vi "DG Measure.vi"(5 "PJVS setup":T2={"PJVS type"=enum."AC-supraVOLTcontrol", "Status Refnum"=refnum, "AC-supraVOLTcontrol"={"IP address:port (0.0.0.0:0000)"="0.0.0.0:0000", "Timeouts"={"TCP Read & Write (ms)"=7000, "Sensors readout"=5000, "PJVS setup"=10000, "Nullmeter readout"=5000, "Multiplexer setup"=3000, "57XX setup"=15000, "Generator setup"=5000, "Synthesizer setup"=3000, "Sampler readout"=10000}, "Simulation mode"=FALSE, "Debug mode"=FALSE}, "NPL bias source"={"DataSocketCluster"={"Server Machine"="CZC", "Client Machine"="localhost", "Data"="P2", "TimeStamp"=0.0, "Count"=1, "Target Process"="General Server"}}, "Manual PJVS"={"PJVS frequency (Hz)"=0.0, "Reference voltages (V)"=[], "File with PJVS voltages"=path ""}, "VTT PJVS"={"some VTT only property"=""}} {"NPL bias source"."DataSocketCluster"."TimeStamp" format="%.2f"}, 8 "error in":errorcluster, 9 "DG measurement":T1={"Signal frequencies (Hz)"=[1000.0], "Signal amplitudes (V)"=[0.707], "Sampling frequencies (Hz)"=[10000000.0], "Record lengths (multiples of periods)"=[10000.0], "Calculate results"=FALSE, "Algorithm"="TWM-PJVSSubS", "TWM data directories"=[], "TWM data directories relative"=[], "PJVS frequencies (Hz)"=[1000.0], "PJVS reference voltages array of vector cluster"=[], "Requested PJVS steps"=[20], "Data folder"=path "", "Rs"=0, "Re"=0, "Settle down after PJVS change (s)"=1.0, "Switch position"=0.0, "PJVS amplitudes (Hz)"=[1000.0], "DG measurement info files"=[]} {"PJVS amplitudes (Hz)" format="%#_3p"; "PJVS reference voltages array of vector cluster"."PJVS reference voltages vector" format="%#_3p"; "PJVS frequencies (Hz)" format="%#_3p"; "Record lengths (multiples of periods)" format="%#_3p"; "Sampling frequencies (Hz)" format="%#_3p"; "Signal amplitudes (V)" format="%#_3p"; "Signal frequencies (Hz)" format="%#_3p"}, 11 "Common properties":T6={"Measurement status ref"=refnum, "TWM Status ref"=refnum, "Abort ref"=refnum, "Skip waiting ref"=refnum, "GNU Octave path"=path "C:/Program Files/GNU Octave/Octave-6.2.0/mingw64/bin", "TWM+QWTB path"=path "C:/Users/labina/Desktop/TWM-1.8.7.0-full/octprog", "lvlib path"=path "D:/martin/WAC/WACsw - github/control_software/Filter function meter/external libraries/GOLPI 0.7.3.1 source distribution LV 20.0 32 bit/lv_proc.dll", "TWM pipe"="\\\\.\\pipe\\TWM:server", "PJVS status ref"=refnum, "WAC path"=path ""}) -> (0 "error out":errorcluster)   [LabVIEW 2020]
doc: "Main VI to run cable error measurement. Setup devices, run loop for all freuencies, stop devices."
uses:
  external libraries/varilib/varilib.lvlib
  external libraries/TWM-1.8.7.0-client/TWM Client.lvlib
  <vilib>/Utility/error.llb/DialogType.ctl
  Utilities/Type definitions/Common properties.ctl
  General PJVS driver/Type definitions/PJVS Type.ctl
  external libraries/acsvcontrol-driver/Public/Type Definitions/Timeouts.ctl
  external libraries/acsvcontrol-driver/ACSVcontrol-driver.lvlib
  external libraries/JV modified NPL Bias source/DataSocketCluster external.ctl
  General PJVS driver/Type definitions/PJVS.ctl
  DG measurement.ctl
panel:
  out "last PJVS set frequency":dbl
  out "last set PJVS steps":u32
  out "last PJVS reference voltages":dbl[](array[numeric])
  out "previous PJVS steps":u32=2147483647
  out "previous PJVS amplitude":dbl=nan format="%#_13g"
  out "previous PJVS frequency":dbl=nan format="%#_13g"
  out "TWM handle":i32
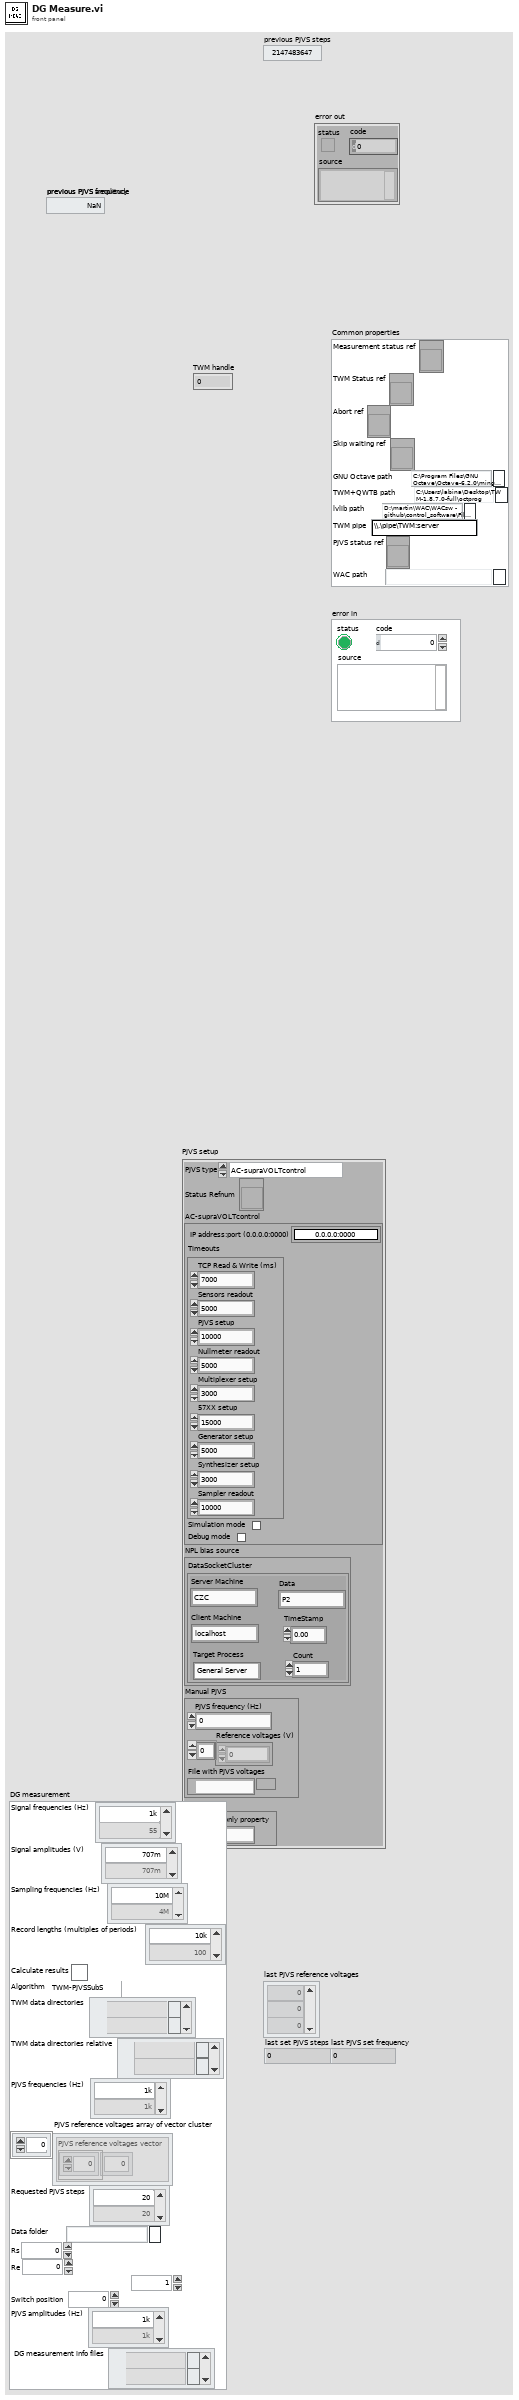
[diagram p1: front panel]
types:
  T1 = typedef "DG measurement.ctl" = cluster{"Signal frequencies (Hz)":dbl[], "Signal amplitudes (V)":dbl[], "Sampling frequencies (Hz)":dbl[], "Record lengths (multiples of periods)":dbl[], "Calculate results":bool, "Algorithm":string, "TWM data directories":path[], "TWM data directories relative":path[], "PJVS frequencies (Hz)":dbl[], "PJVS reference voltages array of vector cluster":cluster{"PJVS reference voltages vector":dbl[]}[], "Requested PJVS steps":u32[], "Data folder":path, "Rs":i32, "Re":i32, "Settle down after PJVS change (s)":dbl, "Switch position":dbl, "PJVS amplitudes (Hz)":dbl[], "DG measurement info files":path[]}
  T2 = typedef "PJVS.ctl" = cluster{"PJVS type":T3, "Status Refnum":refnum<vi>, "AC-supraVOLTcontrol":cluster{"IP address:port (0.0.0.0:0000)":string, "Timeouts":T4, "Simulation mode":bool, "Debug mode":bool}, "NPL bias source":cluster{"DataSocketCluster":T5}, "Manual PJVS":cluster{"PJVS frequency (Hz)":dbl, "Reference voltages (V)":dbl[], "File with PJVS voltages":path}, "VTT PJVS":cluster{"some VTT only property":string}}
  T3 = typedef "PJVS Type.ctl" = enum16{"AC-supraVOLTcontrol", "JV modified NPL bias control", "Manual PJVS", "VTT PJVS"}
  T4 = typedef "ACSVcontrol-driver.lvlib/Timeouts.ctl" = cluster{"TCP Read & Write (ms)":i32, "Sensors readout":i32, "PJVS setup":i32, "Nullmeter readout":i32, "Multiplexer setup":i32, "57XX setup":i32, "Generator setup":i32, "Synthesizer setup":i32, "Sampler readout":i32}
  T5 = typedef "DataSocketCluster external.ctl" = cluster{"Server Machine":string, "Client Machine":string, "Data":string, "TimeStamp":dbl, "Count":i32, "Target Process":string}
  T6 = typedef "Common properties.ctl" = cluster{"Measurement status ref":refnum<vi>, "TWM Status ref":refnum<vi>, "Abort ref":refnum<vi>, "Skip waiting ref":refnum<vi>, "GNU Octave path":path, "TWM+QWTB path":path, "lvlib path":path, "TWM pipe":string, "PJVS status ref":refnum<vi>, "WAC path":path}
  T7 = typedef "DialogType.ctl" = u16
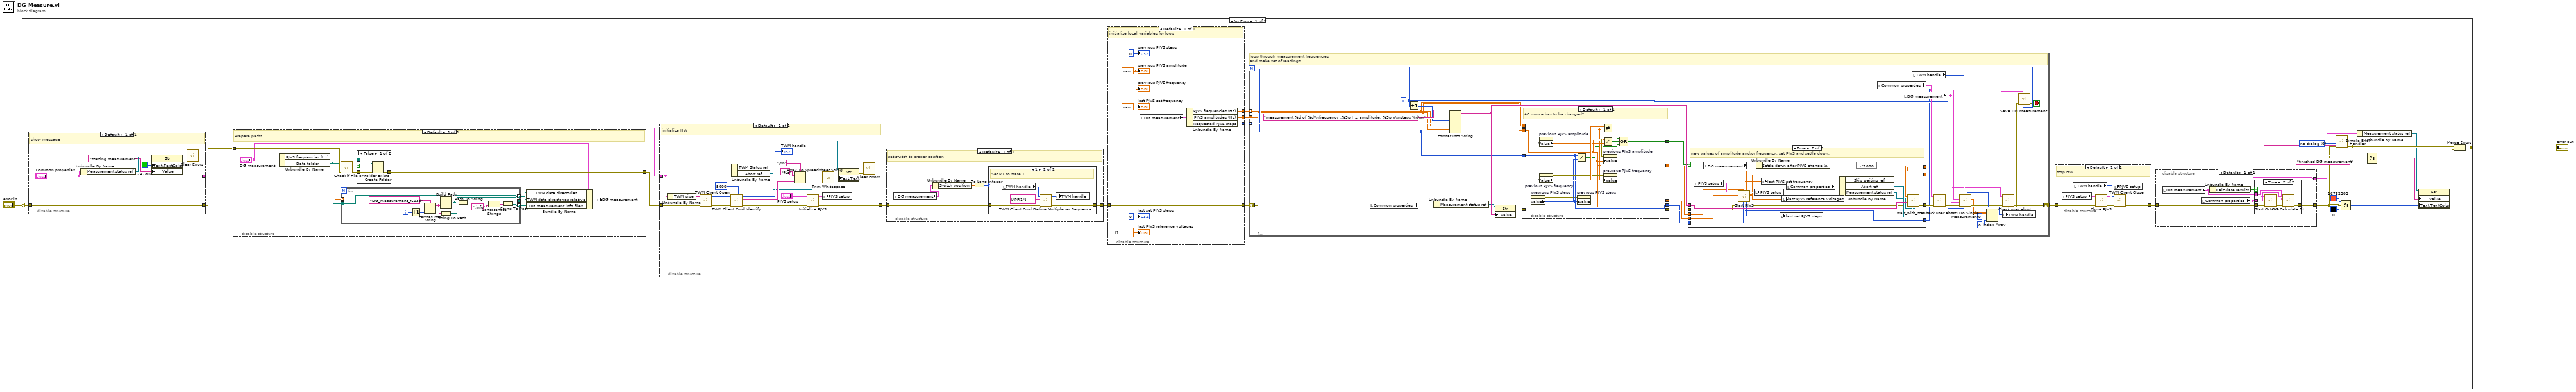
[diagram p0: block diagram]
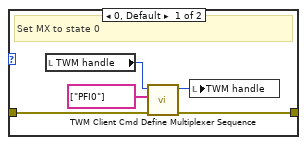
[diagram p3: hidden frame]
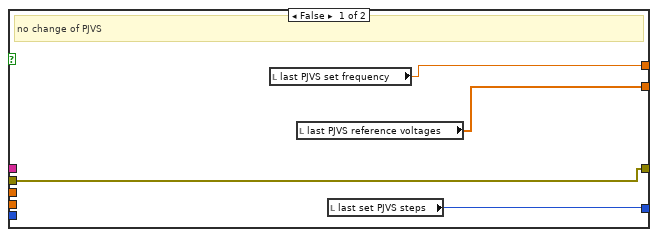
[diagram p5: hidden frame]
diagram:
  n1 = case shown="No Error" "error in" {
    selector: "error in" -> [w8 w188]
    tunnel: [w14 w188] -> w2
    frame No Error {
      w16 = T7 0 items=["no dialog", "OK message", "continue or stop message", "OK message + warnings", "continue/stop + warnings"] ("type of dialog (OK msg:1)")
      n2 = disable-structure shown="Default" {
        disable-tunnel: w8 -> [w91]
        disable-tunnel: [w91] -> w4
        disable-tunnel: ["Common properties"] -> w26
        frame Enabled {
          # "show message"
          n3 = Unbundle By Name("Common properties") -> ("Measurement status ref"=w94:refnum<vi>)
          n4 = property class="Str"(reference=w94, "Text.TextColor"=u32 247808 ("Text.Text Colors:Text Color"), "Value"="starting measurement") -> (error out=w95:errorcluster)  [unwired: 1 in, 1 out]
          n5 = call <vilib>:"Clear Errors.vi"("error in (no error)"=w95) -> ()  [unwired: 5 in, 2 out]
        }
      }
      n6 = disable-structure shown="Default" {
        disable-tunnel: w4 -> [w36]
        disable-tunnel: [w35] -> w3
        frame Enabled {
          # "Prepare paths"
          n7 = Unbundle By Name("DG measurement") -> ("PJVS frequencies (Hz)"=w30:dbl[], "Data folder"=w31:path)
          n8 = call <vilib>:"Check if File or Folder Exists.vi"("error in (no error)"=w36, "path"=w31) -> ("error out"=w37:errorcluster, "file or folder exists?"=w38:bool)  [unwired: 7 in, 1 out]
          n9 = for {
            tunnel: w31 -> [w49]
            tunnel: [w41] -> w34 mode=indexing
            tunnel: w30 -> [_] mode=indexing
            tunnel: [w44] -> w33 mode=indexing
            tunnel: [w39] -> w32 mode=indexing
            i -> [w47]
            n10 = Increment(x=w47) -> (x+1=w46:i32)
            n11 = Format Into String(format string="DG_measurement_%03d" ("string"), w46) -> (resulting string=w45:string)  [unwired: 2 in, 1 out]
            n12 = String To Path(string=w45) -> (path=w44:path)
            n13 = Build Path(base path=w49, name or relative path=w45) -> (appended path=w41:path)
            n14 = Path To String(path=w41) -> (string=w40:string)
            n15 = Concatenate Strings(w40, ".info" ("string")) -> (w43:string)
            n16 = String To Path(string=w43) -> (path=w39:path)
          }
          n17 = case shown="False" w38 {
            tunnel: w31 -> [w52 _]
            tunnel: [w51 w53] -> w35
            tunnel: w37 -> [w50 w53]
            frame False {
              n18 = Create Folder(path (use dialog)=w52, error in=w50) -> (error out=w51:errorcluster)  [unwired: 1 in, 2 out]
            }
            frame True {
            }
          }
          n19 = Bundle By Name(cluster="DG measurement", "TWM data directories"=w34, "TWM data directories relative"=w33, "DG measurement info files"=w32) -> (w28:T1)
          n20 = local write "DG measurement"(w28) -> ()
        }
      }
      n21 = disable-structure shown="Default" {
        disable-tunnel: [w173] -> w6
        disable-tunnel: w3 -> [w176]
        disable-tunnel: w26 -> [w177]
        frame Enabled {
          # "initialize HW"
          n22 = Unbundle By Name(w177) -> ("TWM pipe"=w183:string)
          n23 = call "TWM Client Open.vi"("error in"=w176, "pipe name"=w183) -> ("error out"=w186:errorcluster, "handle out"=w187:i32)  [unwired: 8 in]
          n24 = call "TWM Client Cmd Identify.vi"("timeout [ms]"=5000, "error in"=w186, "handle"=w187) -> ("error out"=w182:errorcluster, "channel idns"=w179:string[], "handle out"=→"TWM handle":i32)  [unwired: 5 in, 1 out]
          n25 = Unbundle By Name(w177) -> ("TWM Status ref"=w171:refnum<vi>, "Abort ref"=w174:refnum<vi>)
          n26 = Array To Spreadsheet String(delimiter (Tab)="\r\n", array=w179, 3:"%s" ("format string")) -> (spreadsheet string=w181:string)
          n27 = call "Initialize PJVS.vi"("Abort Refnum"=w174, "error in (no error)"=w182, "PJVS setup"="PJVS setup") -> ("error out"=w173:errorcluster, "PJVS setup out"=w172:T2)  [unwired: 7 in]
          n28 = call <vilib>:"Trim Whitespace.vi"("string"=w181) -> ("trimmed string"=w170:string)  [unwired: 1 in]
          n29 = local write "PJVS setup"(w172) -> ()
          n30 = property class="Str"(reference=w171, "Text.Text"=w170) -> (error out=w169:errorcluster)  [unwired: 1 in, 1 out]
          n31 = call <vilib>:"Clear Errors.vi"("error in (no error)"=w169) -> ()  [unwired: 5 in, 2 out]
        }
      }
      n32 = disable-structure shown="Default" {
        disable-tunnel: w6 -> [w56]
        disable-tunnel: [w55] -> w5
        frame Enabled {
          # "set switch to proper position"
          n33 = local read "DG measurement"() -> (w54:T1)
          n34 = Unbundle By Name(w54) -> ("Switch position"=w57:dbl)
          n35 = To Long Integer(number=w57) -> (32bit integer=w58:i32)
          n36 = case shown="1" w58 {
            tunnel: w56 -> [w60 w65]
            tunnel: [w59 w64] -> w55
            frame 0, Default {
              # "Set MX to state 0"
              n37 = local read "TWM handle"() -> (w62:i32)
              n38 = call "TWM Client Cmd Define Multiplexer Sequence.vi"("error in"=w60, "sequence item strings"=string[] ["PFI0"], "handle"=w62) -> ("error out"=w59:errorcluster, "handle out"=w63:i32)  [unwired: 7 in]
              n39 = local write "TWM handle"(w63) -> ()
            }
            frame 1 {
              # "Set MX to state 1"
              n40 = local read "TWM handle"() -> (w67:i32)
              n41 = call "TWM Client Cmd Define Multiplexer Sequence.vi"("error in"=w65, "sequence item strings"=string[] ["PFI1"], "handle"=w67) -> ("error out"=w64:errorcluster, "handle out"=w68:i32)  [unwired: 7 in]
              n42 = local write "TWM handle"(w68) -> ()
            }
          }
        }
      }
      n43 = disable-structure shown="Default" {
        disable-tunnel: [w89] -> w25
        disable-tunnel: w5 -> [w89]
        disable-tunnel: [w87] -> w10
        disable-tunnel: [w86] -> w9
        disable-tunnel: [w84] -> w7
        frame Enabled {
          w85 = nan ("previous TWM result value")
          # "initialize local variables for loop"
          n44 = local read "DG measurement"() -> (w88:T1)
          n45 = Unbundle By Name(w88) -> ("PJVS frequencies (Hz)"=w87:dbl[], "PJVS amplitudes (Hz)"=w86:dbl[], "Requested PJVS steps"=w84:u32[])
          "previous PJVS frequency" <- w85
          "previous PJVS amplitude" <- w85
          "previous PJVS steps" <- u32 0 ("previous PJVS steps")
          "last PJVS reference voltages" <- dbl[] [] ("last PJVS reference voltages")
          "last set PJVS steps" <- u32 0 ("last set PJVS steps")
          "last PJVS set frequency" <- nan ("last PJVS set frequency")
        }
      }
      n46 = for {
        N -> [w123]
        shift-right: [w104] -> w27
        shift-left: w25 -> [w122]
        tunnel: w10 -> [w100] mode=indexing
        tunnel: w9 -> [w99] mode=indexing
        tunnel: w7 -> [w98] mode=indexing
        i -> [w105]
        stop <- w103 stop-if-true
        # "loop through measurement frequencies\nand make set of readings"
        n47 = local read "Common properties"() -> (w120:T6)
        n48 = Increment(x=w105) -> (x+1=w112:i32)
        n49 = Unbundle By Name(w120) -> ("Measurement status ref"=w121:refnum<vi>)
        n50 = Format Into String(format string="measurement %d of %d\\nfrequency :%3p Hz, amplitude: %3p V\\nsteps %d\\n", w112, w123, w100, w99, w98) -> (resulting string=w124:string)  [unwired: 2 in, 1 out]
        n51 = property class="Str"(reference=w121, error in=w122, "Value"=w124) -> (error out=w118:errorcluster)  [unwired: 1 out]
        n52 = disable-structure shown="Default" {
          disable-tunnel: w99 -> [w131]
          disable-tunnel: w100 -> [w130]
          disable-tunnel: [w137] -> w101
          disable-tunnel: w118 -> [w137]
          disable-tunnel: [w134] -> w119
          disable-tunnel: [w131] -> w117
          disable-tunnel: [w130] -> w116
          disable-tunnel: w98 -> [w127]
          disable-tunnel: [w127] -> w96
          frame Enabled {
            # "AC source has to be changed?"
            n53 = property on="previous PJVS steps" class="DigNum (strict)"() -> (error out=w126:errorcluster, "Value"=w128:u32)  [unwired: 2 in, 1 out]
            n54 = property on="previous PJVS amplitude" class="DigNum (strict)"() -> (error out=w133:errorcluster, "Value"=w138:dbl)  [unwired: 2 in, 1 out]
            n55 = property on="previous PJVS frequency" class="DigNum (strict)"() -> (error out=w132:errorcluster, "Value"=w139:dbl)  [unwired: 2 in, 1 out]
            n56 = Not Equal?(x=w127, y=w128) -> (x != y?=w129:bool)
            n57 = property on="previous PJVS steps" class="DigNum (strict)"(error in=w126, "Value"=w127) -> ()  [unwired: 1 in, 2 out]
            n58 = Not Equal?(x=w139, y=w130) -> (x != y?=w135:bool)
            n59 = Not Equal?(x=w131, y=w138) -> (x != y?=w136:bool)
            n60 = property on="previous PJVS amplitude" class="DigNum (strict)"(error in=w133, "Value"=w131) -> ()  [unwired: 1 in, 2 out]
            n61 = property on="previous PJVS frequency" class="DigNum (strict)"(error in=w132, "Value"=w130) -> ()  [unwired: 1 in, 2 out]
            n62 = Compound Arithmetic op=OR(w135, w136, w129) -> (w134:bool)
          }
        }
        n63 = case shown="True" w119 {
          tunnel: w124 -> [_ w162]
          tunnel: [w143 w161] -> w115
          tunnel: w101 -> [w143 w152]
          tunnel: w117 -> [_ w145]
          tunnel: w116 -> [_ w146]
          tunnel: [w142 w149] -> w97
          tunnel: [w141 w148] -> _
          tunnel: [w140 w147] -> _
          tunnel: w96 -> [_ w144]
          frame False {
            # "no change of PJVS"
            n64 = local read "last PJVS set frequency"() -> (w140:dbl)
            n65 = local read "last PJVS reference voltages"() -> (w141:dbl[])
            n66 = local read "last set PJVS steps"() -> (w142:u32)
          }
          frame True {
            # "new values of amplitude and/or frequency, set PJVS and settle down."
            n67 = local read "PJVS setup"() -> (w150:T2)
            n68 = local read "DG measurement"() -> (w154:T1)
            n69 = call "Start PJVS.vi"("Requiested PJVS steps"=w144, "Requested PJVS frequency (Hz)"=w146, "error in (pass through)"=w152, "Maximal signal amplitude (V)"=w145, "PJVS setup"=w150) -> ("error out"=w151:errorcluster, "PJVS reference voltages (1 period, V)"=w148:dbl[], "PJVS setup out"=w153:T2, "Set PJVS steps"=w149:u32, "Set frequency (Hz)"=w147:dbl)  [unwired: 2 in]
            n70 = local write "PJVS setup"(w153) -> ()
            n71 = Unbundle By Name(w154) -> ("Settle down after PJVS change (s)"=w159:dbl)
            n72 = local write "last PJVS set frequency"(w147) -> ()
            n73 = local write "last set PJVS steps"(w149) -> ()
            n74 = local write "last PJVS reference voltages"(w148) -> ()
            n75 = local read "Common properties"() -> (w158:T6)
            n76 = Unbundle By Name(w158) -> ("Skip waiting ref"=w157:refnum<vi>, "Abort ref"=w156:refnum<vi>, "Measurement status ref"=w155:refnum<vi>)
            n77 = expression code="x*1000"(w159) -> (w160:dbl)
            n78 = call "wait_with_status.vi"("stat ref"=w155, "stop ref"=w156, "second stop ref"=w157, "error in"=w151, "comment"=w162, "ms to wait"=w160) -> ("error out"=w161:errorcluster)  [unwired: 4 in, 1 out]
          }
        }
        n79 = local read "Common properties"() -> (w109:T6)
        n80 = local read "DG measurement"() -> (w102:T1)
        n81 = local read "TWM handle"() -> (w111:i32)
        n82 = call "Check user abort.vi"("error in (no error)"=w115, "Common properties"=w109) -> ("error out"=w107:errorcluster)  [unwired: 9 in]
        n83 = call "DG Do Single Measurement.vi"("Iteration index"=w105, "TWM handle in"=w111, "error in (no error)"=w107, "DG measurement"=w102, "Common properties"=w109) -> ("error out"=w108:errorcluster, "TWM result as number"=w106:dbl[][], "TWM handle out"=w110:i32)  [unwired: 4 in]
        n84 = Index Array(array=w106, index (row)=0, index (col)=0 ("disabled index (col)")) -> ()  [unwired: 1 out]
        n85 = call "Check user abort.vi"("error in (no error)"=w108, "Common properties"=w109) -> ("error out"=w104:errorcluster)  [unwired: 9 in]
        n86 = local write "TWM handle"(w110) -> ()
        n87 = call "Save DG measurement.vi"("Index"=w105, "DG measurement"=w102, "error in"=w104, "Set PJVS steps"=w97) -> ("error out"=w103:errorcluster)  [unwired: 7 in]
      }
      n88 = disable-structure shown="Default" {
        disable-tunnel: w27 -> [w167]
        disable-tunnel: [w163] -> w13
        frame Enabled {
          # "stop HW"
          n89 = local read "PJVS setup"() -> (w166:T2)
          n90 = local read "TWM handle"() -> (w168:i32)
          n91 = call "Close PJVS.vi"("error in (pass through)"=w167, "PJVS setup"=w166) -> ("error out"=w164:errorcluster, "PJVS setup out"=w165:T2)  [unwired: 8 in]
          n92 = local write "PJVS setup"(w165) -> ()
          n93 = call "TWM Client Close.vi"("error in"=w164, "handle in"=w168) -> ("error out"=w163:errorcluster)  [unwired: 9 in]
        }
      }
      n94 = disable-structure shown="Default" {
        disable-tunnel: w13 -> [w73]
        disable-tunnel: [w72] -> w12
        disable-tunnel: [w69] -> w11
        frame Enabled {
          n95 = local read "DG measurement"() -> (w71:T1)
          n96 = local read "Common properties"() -> (w69:T6)
          n97 = Unbundle By Name(w71) -> ("Calculate results"=w70:bool)
          n98 = case shown="True" w70 {
            tunnel: w73 -> [w74 w79]
            tunnel: [w74 w77] -> w72
            tunnel: w71 -> [_ w75]
            tunnel: w69 -> [_ w76]
            frame False {
            }
            frame True {
              n99 = call "Start Octave.vi"("error in (no error)"=w79, "Common properties"=w76) -> ("error out"=w78:errorcluster)  [unwired: 9 in]
              n100 = call "DG Calculate Fit.vi"("error in (no error)"=w78, "DG measurement"=w75, "Common properties"=w76) -> ("error out"=w77:errorcluster)  [unwired: 8 in]
            }
          }
        }
      }
      n101 = call <vilib>:"Simple Error Handler.vi"("type of dialog (OK msg:1)"=w16, "error in (no error)"=w12) -> ("error out"=w20:errorcluster, "message"=w24:string)  [unwired: 3 in, 3 out]
      n102 = Select(t=u32 16732202 ("Text.Text Colors:Text Color"), s=w12, f=u32 0 ("Text.Text Colors:Text Color")) -> (s? t:f=w22:u32)
      n103 = Unbundle By Name(w11) -> ("Measurement status ref"=w19:refnum<vi>)
      n104 = Select(t=w24, s=w20, f="finished DG measurement") -> (s? t:f=w23:string)
      n105 = property class="Str"(reference=w19, "Value"=w23, "Text.TextColor"=w22) -> (error out=w21:errorcluster)  [unwired: 1 in, 1 out]
      n106 = Merge Errors(w20, w21) -> (w14:errorcluster)
    }
    frame Error {
    }
  }
  "error out" <- w2
